vi "Format String To Numeric Info.vi"(11 "Format String":string) -> (3 "Numeric Format & Precision Info":T1)   [LabVIEW 2018, in "Numeric Data Type.lvclass"]
uses:
  Numeric Data Type.lvclass
  Numeric Info.ctl
  Numeric Format Enum.ctl
  Precision Type.ctl
  Padding.ctl
  <resource>/PropertyPages/Pages/pp_Numeric_Formats.ctl
  Justify Padding Enum.ctl
panel:
  # "0 = <no modifiers>\n1 = -\n2 = 0"
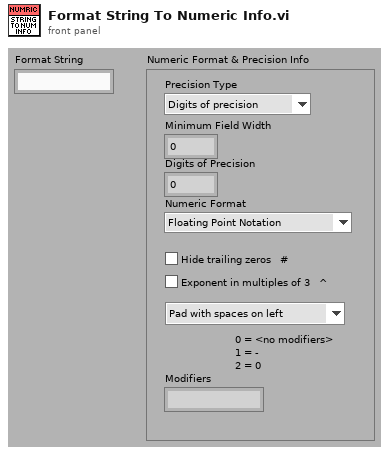
[diagram p1: front panel]
types:
  T1 = typedef "Numeric Data Type.lvclass/Numeric Info.ctl" = cluster{"Minimum Field Width":i32, "Digits of Precision":i32, "Numeric Format":T2, "Precision Type":T3, "Hide trailing zeros":bool, "exponent":bool, "just/pad":T4, "Modifiers":string}
  T2 = typedef "Numeric Data Type.lvclass/Numeric Format Enum.ctl" = enum16{"Floating Point Notation", "Scientific Notation", "Engineering Notation", "SI Notation", "<not used>", "Decimal", "Hexadecimal", "Octal", "Binary", "<not used 2>", "Absolute Time", "Relative Time"}
  T3 = typedef "Numeric Data Type.lvclass/Precision Type.ctl" = enum16{"Digits of precision", "Significant digits"}
  T4 = typedef "Numeric Data Type.lvclass/Padding.ctl" = enum16{"Pad with spaces on left", "Pad with spaces on right", "Pad with zeros on left"}
  T5 = typedef "Numeric Data Type.lvclass/Justify Padding Enum.ctl" = enum16{"Pad with spaces on left", "Pad with spaces on right", "Pad with zeros on left"}
  T6 = typedef "pp_Numeric_Formats.ctl" = string[]
  T7 = typedef "Numeric Data Type.lvclass/Format Code.ctl" = cluster{"Code Char":string, "Precision":i32, "MinWidth":u16, "EmbeddedString":string, "Modifiers":string}
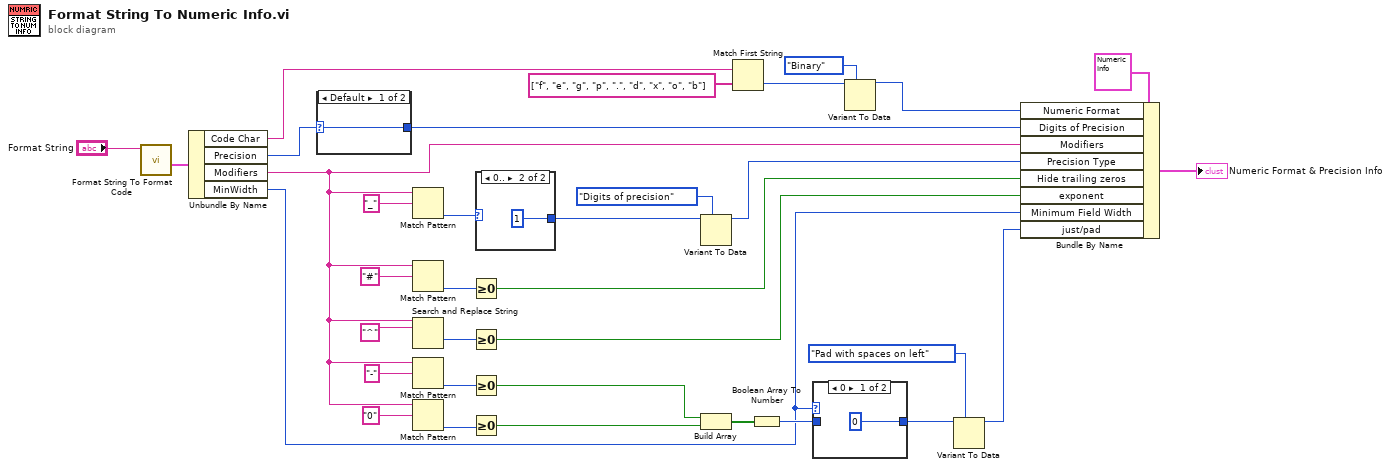
[diagram p0: block diagram]
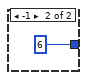
[diagram p2: hidden frame]
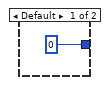
[diagram p3: hidden frame]
diagram:
  n1 = call "Format String To Format Code.vi"("Start String"="Format String") -> ("Format Code"=w11:T7)  [unwired: 7 in, 3 out]
  n2 = Unbundle By Name(w11) -> ("Code Char"=w35:string, "Precision"=w21:i32, "Modifiers"=w7:string, "MinWidth"=w8:u16)
  n3 = case shown="Default" w21 {
    selector: w21 -> [w36 _]
    tunnel: [w36 6] -> w18
    frame Default {
    }
    frame -1 {
    }
  }
  n4 = Match Pattern(string=w7, regular expression="_") -> (offset past match=w33:i32)  [unwired: 1 in, 3 out]
  n5 = Match Pattern(string=w7, regular expression="#") -> (offset past match=w31:i32)  [unwired: 1 in, 3 out]
  n6 = Search and Replace String(input string=w7, search string="^") -> (offset past replacement=w24:i32)  [unwired: 6 in, 3 out]
  n7 = Match Pattern(string=w7, regular expression="-") -> (offset past match=w28:i32)  [unwired: 1 in, 3 out]
  n8 = Match Pattern(string=w7, regular expression="0") -> (offset past match=w27:i32)  [unwired: 1 in, 3 out]
  n9 = Greater Or Equal To 0?(x=w31) -> (x >= 0?=w16:bool)
  n10 = Greater Or Equal To 0?(x=w24) -> (x >= 0?=w15:bool)
  n11 = Greater Or Equal To 0?(x=w28) -> (x >= 0?=w22:bool)
  n12 = Greater Or Equal To 0?(x=w27) -> (x >= 0?=w23:bool)
  n13 = case shown="0.." w33 {
    tunnel: [0 1] -> w17
    frame Default {
    }
    frame 0.. {
    }
  }
  n14 = Variant To Data(type=Precision_Type."Digits of precision" ("Precision Type"), Variant=w17) -> (data=w9:T3)  [unwired: 1 in, 1 out]
  n15 = Build Array(w22, w23) -> (w26:bool[])
  n16 = Match First String(2:T6 ["f", "e", "g", "p", ".", "d", "x", "o", "b"] ("formats"), 3:w35) -> (0:w3:i32)  [unwired: 1 out]
  n17 = Boolean Array To Number(Boolean array=w26) -> (number=w19:u32)
  n18 = case shown="0" w8 {
    tunnel: w19 -> [_ w41]
    tunnel: [u32 0 w41] -> w6
    frame 0 {
    }
    frame Default {
    }
  }
  n19 = Variant To Data(type=Numeric_Format_Enum."Binary", Variant=w3) -> (data=w2:T2)  [unwired: 1 in, 1 out]
  n20 = Variant To Data(type=Justify_Padding_Enum."Pad with spaces on left" ("just/pad"), Variant=w6) -> (data=w4:T5)  [unwired: 1 in, 1 out]
  n21 = Bundle By Name(cluster=T1 {"Minimum Field Width"=0, "Digits of Precision"=0, "Numeric Format"=enum."Floating Point Notation", "Precision Type"=enum."Digits of precision", "Hide trailing zeros"=FALSE, "exponent"=FALSE, "just/pad"=enum."Pad with spaces on left", "Modifiers"=""} ("Numeric Format & Precision Info"), "Numeric Format"=w2, "Digits of Precision"=w18, "Modifiers"=w7, "Precision Type"=w9, "Hide trailing zeros"=w16, "exponent"=w15, "Minimum Field Width"=w8, "just/pad"=w4) -> (→"Numeric Format & Precision Info":T1)
